vi "Profile Status.vi"(8 "error in (no error)":errorcluster, 11 "F4T in":refnum<class "F4T.lvclass">) -> (0 "error out":errorcluster, 2 "Status":T1={"Profile Status"={"Profile State"=enum."Not Running", "Current Profile"=0, "Total Time Remaining"=0, "Total Steps"=0}, "Step Status"={"Current Step"=0, "Step Type"=enum."Instant Change", "Time Remaining"=0}}, 3 "F4T out":refnum<class "F4T.lvclass">)   [LabVIEW 2018, in "F4T.lvlib" / "F4T.lvclass"]
doc: "This Override is used to read a Profile Status."
uses:
  F4T.lvclass
  PPLs/Temp Chamber/Parent/Temp Chamber.lvlibp/Custom Controls/Status.ctl
  PPLs/Temp Chamber/Parent/Temp Chamber.lvlibp/Custom Controls/Profile Status.ctl
  PPLs/Temp Chamber/Parent/Temp Chamber.lvlibp/Custom Controls/Profile State.ctl
  PPLs/Temp Chamber/Parent/Temp Chamber.lvlibp/Custom Controls/Step Status.ctl
  PPLs/Temp Chamber/Parent/Temp Chamber.lvlibp/Custom Controls/Step Type.ctl
  Custom Controls/Command Data.ctl
  PPLs/Temp Chamber/Parent/Temp Chamber.lvlibp/Temp Chamber.lvclass
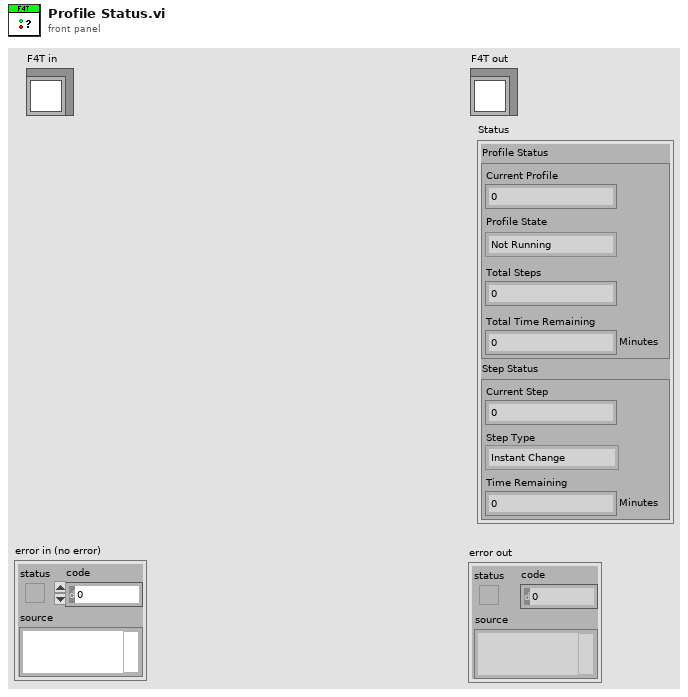
[diagram p1: front panel]
types:
  T1 = typedef "Temp Chamber.lvlibp/Temp Chamber.lvclass/Status.ctl" = cluster{"Profile Status":T2, "Step Status":T4}
  T2 = typedef "Temp Chamber.lvlibp/Temp Chamber.lvclass/Profile Status.ctl" = cluster{"Profile State":T3, "Current Profile":u32, "Total Time Remaining":u32, "Total Steps":u32}
  T3 = typedef "Temp Chamber.lvlibp/Temp Chamber.lvclass/Profile State.ctl" = enum16{"Running", "Not Running", "Paused", "Completed", "Terminated"}
  T4 = typedef "Temp Chamber.lvlibp/Temp Chamber.lvclass/Step Status.ctl" = cluster{"Current Step":u32, "Step Type":T5, "Time Remaining":u32}
  T5 = typedef "Temp Chamber.lvlibp/Temp Chamber.lvclass/Step Type.ctl" = enum16{"Instant Change", "Wait For", "Jump", "Soak", "Ramp Rate", "Ramp Time", "End", "Other"}
  T6 = typedef "F4T.lvlib/F4T.lvclass/Command Data.ctl" = cluster{"ParameterID":u32, "InstanceId":u32, "Value":string}
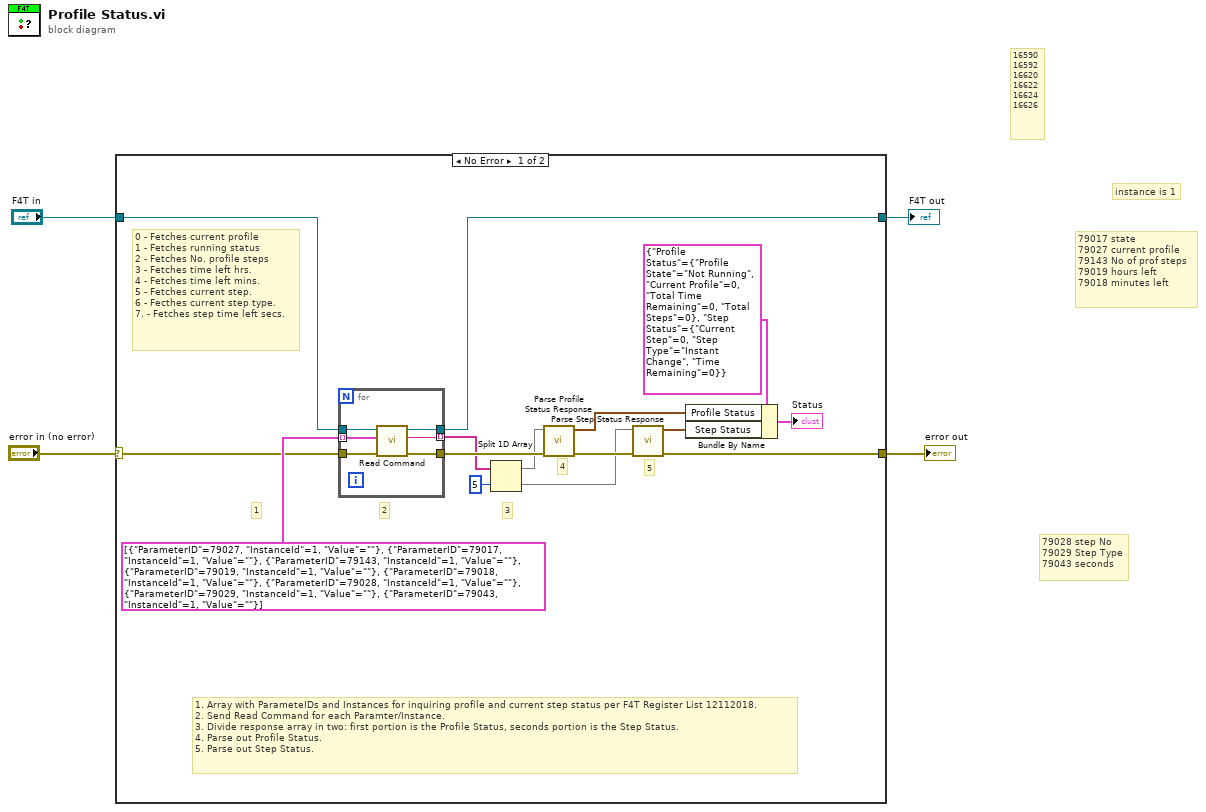
[diagram p0: block diagram]
diagram:
  # "79028 step No\n79029 Step Type\n79043 seconds"
  # "16590\n16592\n16620\n16622\n16624\n16626"
  # "instance is 1"
  # "79017 state\n79027 current profile\n79143 No of prof steps\n79019 hours left\n79018 minutes left"
  n1 = case shown="No Error" "error in (no error)" {
    selector: "error in (no error)" -> [w16 w27]
    tunnel: [w7 w27] -> w3
    tunnel: [w12 w26] -> w1
    tunnel: "F4T in" -> [w13 w26]
    frame No Error {
      # "0 - Fetches current profile\n1 - Fetches running status\n2 - Fetches No. profile steps\n3 - Fetches time left hrs.\n4 - Fetches time left mins.\n5 - Fetches current step.\n6 - Fecthes current step type.\n7. - Fetches step time left secs."
      # "1. Array with ParameteIDs and Instances for inquiring profile and current step status per F4T Register List 12112018.\n2. Send Read Command for each Paramter/Instance.\n3. Divide response array in two: first portion is the Profile Status, seconds portion is the Step Status.\n4. Parse out Profile Status.\n5. Parse out Step Status."
      # "5"
      # "4"
      # "3"
      # "2"
      # "1"
      n2 = for {
        tunnel: [w25] -> w11 mode=indexing
        tunnel: T6[] [{"ParameterID"=79027, "InstanceId"=1, "Value"=""}, {"ParameterID"=79017, "InstanceId"=1, "Value"=""}, {"ParameterID"=79143, "InstanceId"=1, "Value"=""}, {"ParameterID"=79019, "InstanceId"=1, "Value"=""}, {"ParameterID"=79018, "InstanceId"=1, "Value"=""}, {"ParameterID"=79028, "InstanceId"=1, "Value"=""}, {"ParameterID"=79029, "InstanceId"=1, "Value"=""}, {"ParameterID"=79043, "InstanceId"=1, "Value"=""}] -> [w24] mode=indexing
        tunnel: w16 -> [w23]
        tunnel: [w22] -> w14
        tunnel: w13 -> [w21]
        tunnel: [w20] -> w12
        n3 = call "Read Command.vi"("error in (no error)"=w23, "Command Data"=w24, "F4T in"=w21) -> ("error out"=w22:errorcluster, "Response"=w25:string, "F4T out"=w20:refnum<class "F4T.lvclass">)  [unwired: 6 in]
      }
      n4 = Split 1D Array(array=w11, index=5 ("length")) -> (first subarray=w9:string[], second subarray=w6:string[])
      n5 = call "Parse Profile Status Response.vi"("error in (no error)"=w14, "Profile Status"=w9) -> ("error out"=w8:errorcluster, "Profile Status"=w15:T2)  [unwired: 8 in]
      n6 = call "Parse Step Status Response.vi"("error in (no error)"=w8, "Step Status"=w6) -> ("error out"=w7:errorcluster, "Step Status"=w5:T4)  [unwired: 8 in]
      n7 = Bundle By Name(cluster=T1 {"Profile Status"={"Profile State"=enum."Not Running", "Current Profile"=0, "Total Time Remaining"=0, "Total Steps"=0}, "Step Status"={"Current Step"=0, "Step Type"=enum."Instant Change", "Time Remaining"=0}} ("Status"), "Profile Status"=w15, "Step Status"=w5) -> (→"Status":T1)
    }
    frame Error {
    }
  }
  "error out" <- w3
  "F4T out" <- w1
